vi "Begin.vi"(8 "error in":errorcluster) -> (0 "error out":errorcluster)   [LabVIEW 2017]
doc: "Called before other user functions, this VI is expected to open initial I/O refnums, load in file data, and do all program initialization. Notice that the <B>error out</B> terminal is simply used for data flow. Wiring it to other structures or subVIs ensures that this VI runs first."
uses:
  <vilib>/Rock Robotics/WPI/DriverStation/WPI_DriverStationRobotMode2.ctl
  TypeDef/CLUSTER_Arm_Device_IDs.ctl
  TypeDef/CLUSTER_Talon_Setup.ctl
  Public/Documents/Cross The Road Electronics/Phoenix-LabVIEW/Motor Controller/Controls/CTRE_Phoenix_MotorControl_FeedbackDevice.ctl
  TypeDef/CLUSTER_PID.ctl
  Robot Global Data.vi
  Globals/Global_STOP.vi
  Globals/Global_Device_IDs.vi
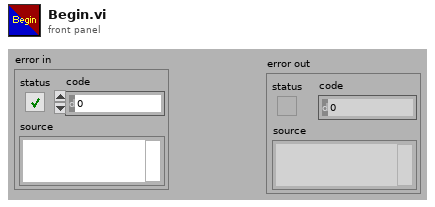
[diagram p1: front panel]
types:
  T1 = typedef "CTRE_Phoenix_MotorControl_FeedbackDevice.ctl" = i8
  T2 = typedef "CLUSTER_Talon_Setup.ctl" = cluster{"Talon SRX ID":u8, "PhaseSensor":bool, "Invert Motor?":bool, "Phoenix Feedback Select":T1, "pidLoopldx":i32, "PID":T3}
  T3 = typedef "CLUSTER_PID.ctl" = cluster{"P":dbl, "I":dbl, "D":dbl, "F":dbl, "I Zone":dbl}
  T4 = typedef "CLUSTER_Arm_Device_IDs.ctl" = cluster{"Elbow Setup":T2, "Telescope Setup":T2, "Wrist Setup":T2}
  T5 = typedef "WPI_DriverStationRobotMode2.ctl" = enum16{"Autonomous Disabled", "Autonomous Enabled", "Teleop Disabled", "Teleop Enabled", "Disconnected", "Finish", "Test Disabled", "Test Enabled", "Emergency Stopped"}
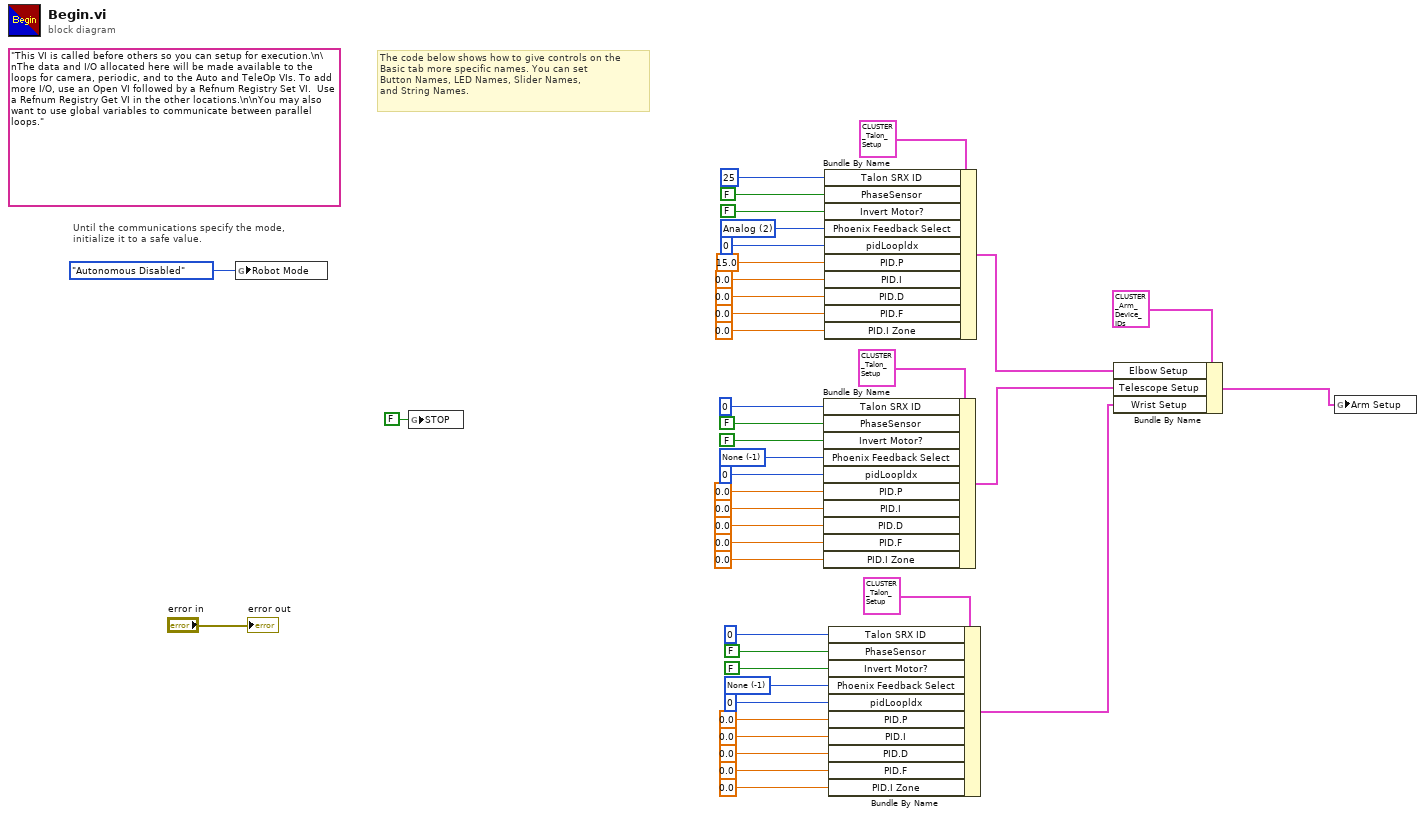
[diagram p0: block diagram]
diagram:
  w8 = T1 -1 items=["None"=-1, "QuadEncoder"=0, "Analog"=2, "Tachometer"=4, "Pulse Width Encoded Position"=8, "Sensor Sum (S0 + S1)"=9, "Sensor Difference (D0 - D1)"=10, "Remote Source 0"=11, "Remote Source 1"=12, "Software Emulated"=15] ("Phoenix Feedback Select")
  w18 = T1 -1 items=["None"=-1, "QuadEncoder"=0, "Analog"=2, "Tachometer"=4, "Pulse Width Encoded Position"=8, "Sensor Sum (S0 + S1)"=9, "Sensor Difference (D0 - D1)"=10, "Remote Source 0"=11, "Remote Source 1"=12, "Software Emulated"=15] ("Phoenix Feedback Select")
  w31 = T1 2 items=["None"=-1, "QuadEncoder"=0, "Analog"=2, "Tachometer"=4, "Pulse Width Encoded Position"=8, "Sensor Sum (S0 + S1)"=9, "Sensor Difference (D0 - D1)"=10, "Remote Source 0"=11, "Remote Source 1"=12, "Software Emulated"=15] ("Phoenix Feedback Select")
  (unwired) "This VI is called before others so you can setup for execution.\n\nThe data and I/O allocated here will be made available to the loops for camera, periodic, and to the Auto and TeleOp VIs. To add more I/O, use an Open VI followed by a Refnum Registry Set VI.  Use a Refnum Registry Get VI in the other locations.\n\nYou may also want to use global variables to communicate between parallel loops."
  # "The code below shows how to give controls on the\nBasic tab more specific names. You can set\nButton Names, LED Names, Slider Names,\nand String Names."
  # "Until the communications specify the mode,\ninitialize it to a safe value."
  n1 = global write "Robot Global Data.vi" "Robot Mode"(WPI_DriverStationRobotMode2."Autonomous Disabled" ("Robot Mode")) -> ()
  n2 = global write "Global_STOP.vi" "STOP"(FALSE ("STOP")) -> ()
  n3 = Bundle By Name(cluster=T2 {"Talon SRX ID"=0, "PhaseSensor"=FALSE, "Invert Motor?"=FALSE, "Phoenix Feedback Select"=-1, "pidLoopldx"=0, "PID"={"P"=0.0, "I"=0.0, "D"=0.0, "F"=0.0, "I Zone"=0.0}} ("Talon Setup"), "Talon SRX ID"=u8 0, "PhaseSensor"=FALSE, "Invert Motor?"=FALSE, "Phoenix Feedback Select"=w18, "pidLoopldx"=0, "PID.P"=0.0, "PID.I"=0.0, "PID.D"=0.0, "PID.F"=0.0, "PID.I Zone"=0.0) -> (w13:T2)
  n4 = Bundle By Name(cluster=T2 {"Talon SRX ID"=0, "PhaseSensor"=FALSE, "Invert Motor?"=FALSE, "Phoenix Feedback Select"=-1, "pidLoopldx"=0, "PID"={"P"=0.0, "I"=0.0, "D"=0.0, "F"=0.0, "I Zone"=0.0}} ("Talon Setup"), "Talon SRX ID"=u8 25, "PhaseSensor"=FALSE, "Invert Motor?"=FALSE, "Phoenix Feedback Select"=w31, "pidLoopldx"=0, "PID.P"=15.0, "PID.I"=0.0, "PID.D"=0.0, "PID.F"=0.0, "PID.I Zone"=0.0) -> (w35:T2)
  n5 = Bundle By Name(cluster=T2 {"Talon SRX ID"=0, "PhaseSensor"=FALSE, "Invert Motor?"=FALSE, "Phoenix Feedback Select"=-1, "pidLoopldx"=0, "PID"={"P"=0.0, "I"=0.0, "D"=0.0, "F"=0.0, "I Zone"=0.0}} ("Talon Setup"), "Talon SRX ID"=u8 0, "PhaseSensor"=FALSE, "Invert Motor?"=FALSE, "Phoenix Feedback Select"=w8, "pidLoopldx"=0, "PID.P"=0.0, "PID.I"=0.0, "PID.D"=0.0, "PID.F"=0.0, "PID.I Zone"=0.0) -> (w1:T2)
  n6 = Bundle By Name(cluster=T4 {"Elbow Setup"={"Talon SRX ID"=0, "PhaseSensor"=FALSE, "Invert Motor?"=FALSE, "Phoenix Feedback Select"=0, "pidLoopldx"=0, "PID"={"P"=0.0, "I"=0.0, "D"=0.0, "F"=0.0, "I Zone"=0.0}}, "Telescope Setup"={"Talon SRX ID"=0, "PhaseSensor"=FALSE, "Invert Motor?"=FALSE, "Phoenix Feedback Select"=-1, "pidLoopldx"=0, "PID"={"P"=0.0, "I"=0.0, "D"=0.0, "F"=0.0, "I Zone"=0.0}}, "Wrist Setup"={"Talon SRX ID"=0, "PhaseSensor"=FALSE, "Invert Motor?"=FALSE, "Phoenix Feedback Select"=-1, "pidLoopldx"=0, "PID"={"P"=0.0, "I"=0.0, "D"=0.0, "F"=0.0, "I Zone"=0.0}}} ("Arm Device IDs"), "Elbow Setup"=w35, "Telescope Setup"=w13, "Wrist Setup"=w1) -> (w37:T4)
  n7 = global write "Global_Device_IDs.vi" "Arm Setup"(w37) -> ()
  "error out" <- "error in"
